vi "Write Panel to INI__ogtk.vi"(5 "float number format (optional)":string, 8 "error in (no error)":errorcluster, 10 "VI ref":refnum<vi>, 11 "refnum":T1) -> (0 "error out":errorcluster, 3 "refnum out":T1)   [LabVIEW 2018]
doc: "Writes the values of the controls on the Front Panel of <B>VI ref</B> to a standard LabVIEW configuration (INI) file as key-value pairs.s\n\nUse this VI in conjunction with the <B>Read Panel from INI</B> from the OpenG Variant Config palette."
uses:
  <vilib>/Utility/config.llb/Config Data RefNum.ctl
  <vilib>/Utility/config.llb/NI_LVConfig.lvlib
panel:
  # "Write Panel to INI.vi\n\nWrites all Front Panel data to INI file.\n\nPlease visit http://www.OpenG.org to learn about the\nOpen Source LabVIEW software movement.\n\nNOTICE -- YOU MUST LEAVE THIS NOTICE IN PLACE.  PER THE TERMS OF THE LICENSE BELOW, YOU MAY SUBLICENSE THIS SOFTWARE \nIN ANY WAY THAT DOES NOT CONFLICT WITH THIS LICENSE.\n\n### BSD License (http://www.opensource.org/licenses/bsd-license.php) Begin ###\n \nCopyright (c) 2002, Jean-Pierre Drolet <drolet_jp@hotmail.com>\n\nAll rights reserved.\n\nRedistribution and use in source and binary forms, with or without modification, are permitted provided that the following conditions are met:\n\n    * Redistributions of source code must retain the above copyright notice, this list of conditions and the following disclaimer.\n    * Redistributions in binary form must reproduce the above copyright notice, this list of conditions and the following disclaimer in the \n       documentation and/or other materials provided with the distribution.\n    * Neither the name of SciWare, James Kring, Inc., nor the names of its contributors may be used to endorse or promote products derived \n       from this software without specific prior written permission.\n\nTHIS SOFTWARE IS PROVIDED BY THE COPYRIGHT HOLDERS AND CONTRIBUTORS \"AS IS\" AND ANY EXPRESS OR IMPLIED WARRANTIES, \nINCLUDING, BUT NOT LIMITED TO, THE IMPLIED WARRANTIES OF MERCHANTABILITY AND FITNESS FOR A PARTICULAR PURPOSE ARE \nDISCLAIMED. IN NO EVENT SHALL THE COPYRIGHT OWNER OR CONTRIBUTORS BE LIABLE FOR ANY DIRECT, INDIRECT, INCIDENTAL,\n SPECIAL, EXEMPLARY, OR CONSEQUENTIAL DAMAGES (INCLUDING, BUT NOT LIMITED TO, PROCUREMENT OF SUBSTITUTE GOODS OR \nSERVICES; LOSS OF USE, DATA, OR PROFITS; OR BUSINESS INTERRUPTION) HOWEVER CAUSED AND ON ANY THEORY OF LIABILITY, \nWHETHER IN CONTRACT, STRICT LIABILITY, OR TORT (INCLUDING NEGLIGENCE OR OTHERWISE) ARISING IN ANY WAY OUT OF THE USE \nOF THIS SOFTWARE, EVEN IF ADVISED OF THE POSSIBILITY OF SUCH DAMAGE.\n\n### BSD License End ###"
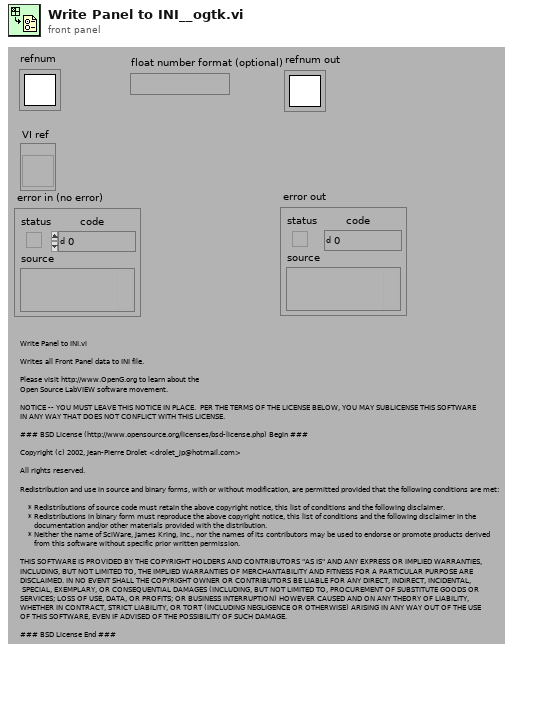
[diagram p1: front panel]
types:
  T1 = typedef "NI_LVConfig.lvlib/Config Data RefNum.ctl" = refnum<k1>
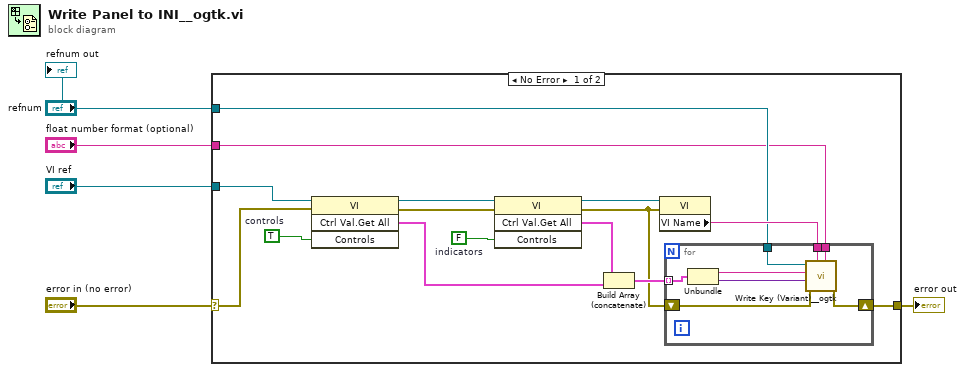
[diagram p0: block diagram]
diagram:
  n1 = case shown="No Error" "error in (no error)" {
    selector: "error in (no error)" -> [w7 w29]
    tunnel: "refnum" -> [w11 _]
    tunnel: [w9 w29] -> w4
    tunnel: "VI ref" -> [w8 _]
    tunnel: "float number format (optional)" -> [w6 _]
    frame No Error {
      w18 = FALSE  # indicators
      w20 = TRUE  # controls
      n2 = invoke class="VI" method="Ctrl Val.Get All"(reference=w8, error in=w7, "Controls"=w20) -> (reference out=w19:refnum<vi>, error out=w14:errorcluster, "Get All Control Values Variant"=w16:cluster{"Name":string, "Variant Data":variant}[])  [unwired: 1 in, 1 out]
      n3 = invoke class="VI" method="Ctrl Val.Get All"(reference=w19, error in=w14, "Controls"=w18) -> (reference out=w15:refnum<vi>, error out=w10:errorcluster, "Get All Control Values Variant"=w17:cluster{"Name":string, "Variant Data":variant}[])  [unwired: 1 in, 1 out]
      n4 = Build Array (concatenate)(w17, w16) -> (w13:cluster{"Name":string, "Variant Data":variant}[])
      n5 = property class="VI"(reference=w15, error in=w10) -> ("VI Name"=w12:string)  [unwired: 2 out]
      n6 = for {
        tunnel: w13 -> [w28] mode=indexing
        tunnel: w12 -> [w27]
        tunnel: w11 -> [w25]
        shift-right: [w24] -> w9
        shift-left: w10 -> [w21]
        tunnel: w6 -> [w23]
        n7 = Unbundle(w28) -> ("Name"=w26:string, "Variant Data"=w22:variant)
        n8 = call <userlib>:"Write Key (Variant)__ogtk.vi"("float number format"=w23, "section"=w27, "error in (no error)"=w21, "key-value"=w22, "key (optional)"=w26, "refnum"=w25) -> ("error out"=w24:errorcluster)  [unwired: 4 in, 1 out]
      }
    }
    frame Error {
    }
  }
  "error out" <- w4
  "refnum out" <- "refnum"
